vi "3_AC_Akım.vi"(10 "Ölçüm Süresi [sn]":i32=60, 11 "Remote IP Address":string="10.1.21.134") -> (0 "error out":errorcluster, 2 "AC AKIM Tüm Fazlar":sgl[][](array[numeric]) format="%.6f")   [LabVIEW 2014]
panel:
  in  "AC Akım FD2 Ic Register":u16=677
  in  "AC Akım FD2 Ib Register":u16=675
  in  "AC Akım FD2 Ia Register":u16=673
  out "AC Akım FD2 Ia":sgl[](array[numeric]) format="%_6f"
  out "AC Akım FD2 Ib":sgl[](array[numeric]) format="%_6f"
  out "AC Akım FD2 Ic":sgl[](array[numeric]) format="%_6f"
  out "AC Akım FD1 Ic":sgl[](array[numeric]) format="%_6f"
  out "AC Akım FD1 Ib":sgl[](array[numeric]) format="%_6f"
  out "AC Akım FD1 Ia":sgl[](array[numeric]) format="%_6f"
  in  "AC Akım FD1 Ic Register":u16=13
  in  "AC Akım FD1 Ib Register":u16=11
  out "Numeric":i32
  in  "AC Akım FD1 Ia Register":u16=9
  out "time stamp":timestamp=timestamp(1426515300 s since 1904-01-01) format="%<%H:%M:%S>T"
  in  "Remote Port":u16=1502
  in  "Stop":bool
  # "MB Ethernet Example Master.vi\n\nInstructions\n1. Run MB Ethernet Example Slave.vi\n2. Run this VI.\n3. Modify the discrete inputs or input registers on the slave -> they're updated on the master.\n4. Modify the coils and registers on the master -> they're updated on the slave."
  # "TCP Parameters"
  # "Slave Read-only Registers"
  # "FD1 Ia"
  # "FD1 Ib"
  # "FD1 Ic"
  # "FD2 Ia"
  # "FD2 Ib"
  # "FD2 Ic"
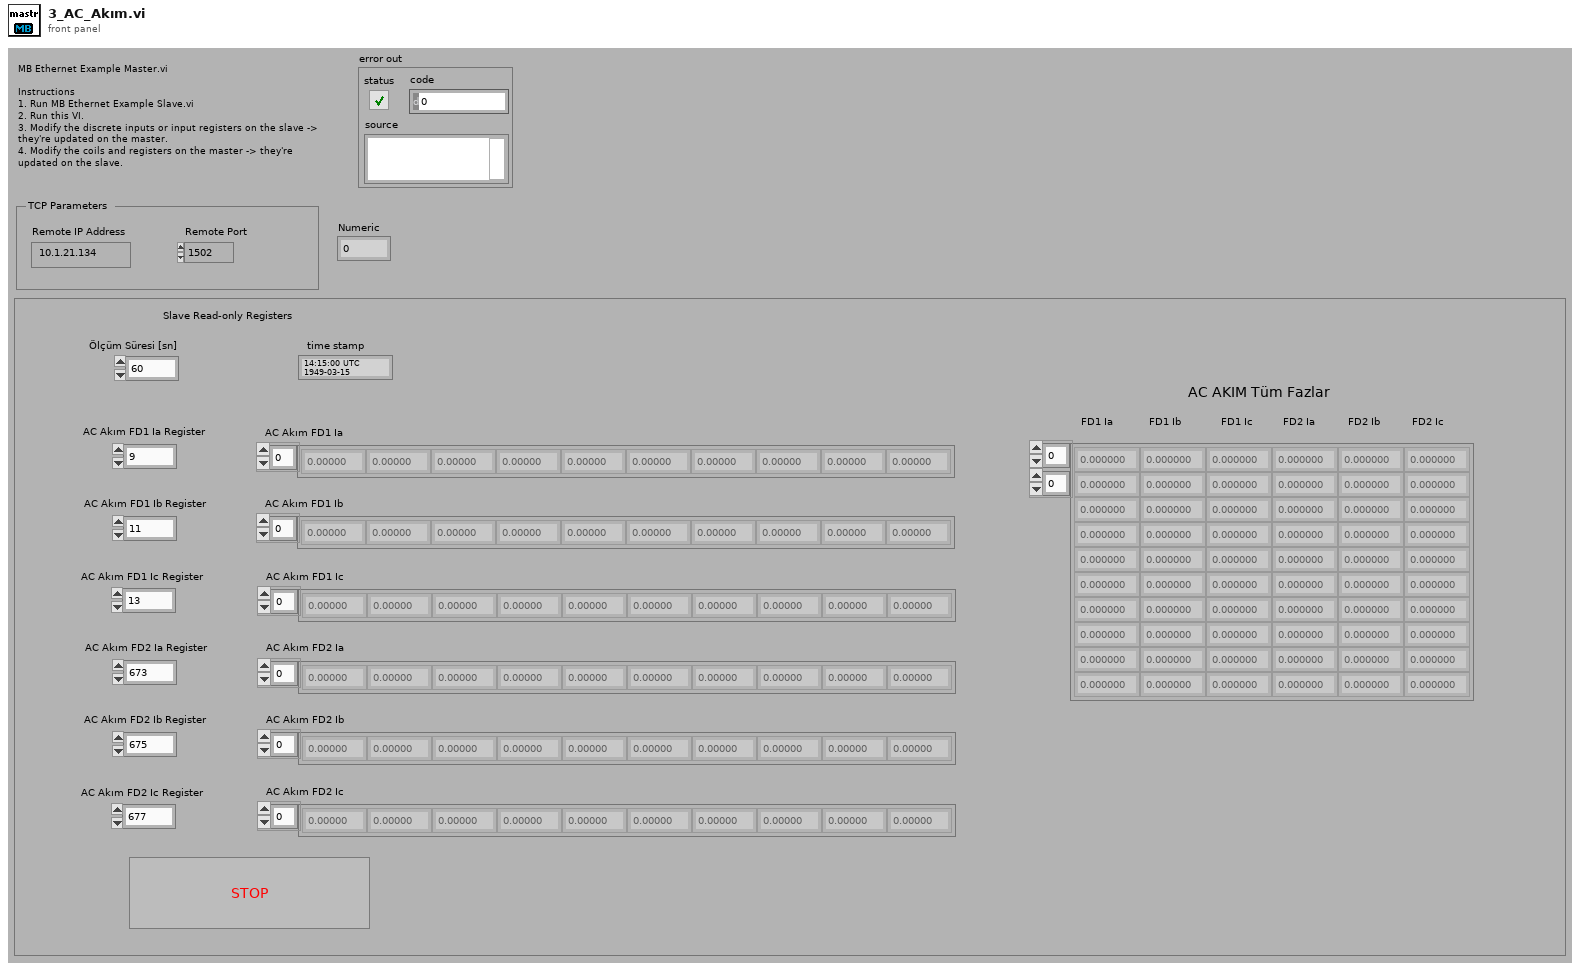
[diagram p1: front panel]
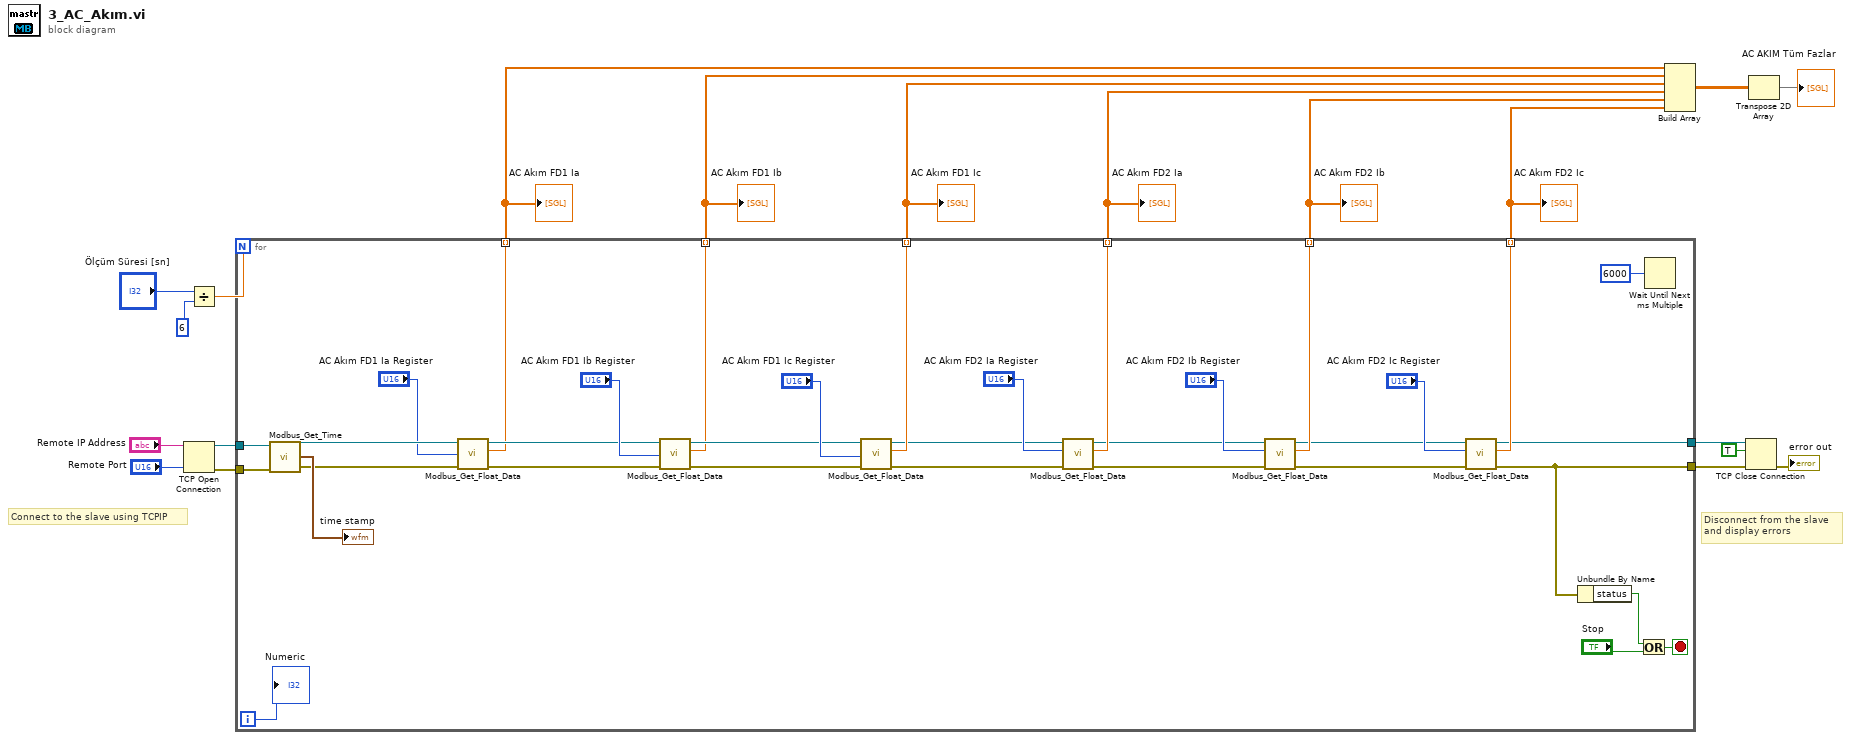
[diagram p0: block diagram]
diagram:
  # "Disconnect from the slave\nand display errors"
  # "Connect to the slave using TCPIP"
  n1 = TCP Open Connection(address="Remote IP Address", remote port or service name="Remote Port") -> (connection ID=w17:refnum<k5>, error out=w16:errorcluster)  [unwired: 1 in, 2 out]
  n2 = Divide(x="Ölçüm Süresi [sn]", y=6) -> (x/y=w12:dbl)
  n3 = for {
    N: w12 -> [_]
    tunnel: [w26] -> w15
    tunnel: w17 -> [w51]
    tunnel: w16 -> [w50]
    tunnel: [w22] -> w9
    tunnel: [w30] -> w8 mode=indexing
    tunnel: [w21] -> w7 mode=indexing
    tunnel: [w37] -> w6 mode=indexing
    tunnel: [w31] -> w5 mode=indexing
    tunnel: [w33] -> w4 mode=indexing
    tunnel: [w32] -> w3 mode=indexing
    i -> [w45]
    stop <- w20 stop-if-true
    n4 = call "Modbus_Get_Time.vi"("error in (no error)"=w50, "TCP Network Connection in"=w51) -> ("error out"=w46:errorcluster, "Time Stamp"=→"time stamp":timestamp, "TCP Network Connection out"=w48:refnum<k5>)  [unwired: 6 in, 1 out]
    n5 = call "Modbus_Get_Float_Data.vi"("error in (no error)"=w46, "Starting Address (2 Bytes)"="AC Akım FD1 Ia Register", "TCP Network Connection in"=w48) -> ("error out"=w42:errorcluster, "Numeric"=w30:sgl, "TCP Network Connection out"=w41:refnum<k5>)  [unwired: 5 in, 1 out]
    n6 = call "Modbus_Get_Float_Data.vi"("error in (no error)"=w42, "Starting Address (2 Bytes)"="AC Akım FD1 Ib Register", "TCP Network Connection in"=w41) -> ("error out"=w39:errorcluster, "Numeric"=w21:sgl, "TCP Network Connection out"=w38:refnum<k5>)  [unwired: 5 in, 1 out]
    n7 = call "Modbus_Get_Float_Data.vi"("error in (no error)"=w39, "Starting Address (2 Bytes)"="AC Akım FD1 Ic Register", "TCP Network Connection in"=w38) -> ("error out"=w29:errorcluster, "Numeric"=w37:sgl, "TCP Network Connection out"=w25:refnum<k5>)  [unwired: 5 in, 1 out]
    n8 = call "Modbus_Get_Float_Data.vi"("error in (no error)"=w29, "Starting Address (2 Bytes)"="AC Akım FD2 Ia Register", "TCP Network Connection in"=w25) -> ("error out"=w28:errorcluster, "Numeric"=w31:sgl, "TCP Network Connection out"=w24:refnum<k5>)  [unwired: 5 in, 1 out]
    n9 = call "Modbus_Get_Float_Data.vi"("error in (no error)"=w28, "Starting Address (2 Bytes)"="AC Akım FD2 Ib Register", "TCP Network Connection in"=w24) -> ("error out"=w27:errorcluster, "Numeric"=w33:sgl, "TCP Network Connection out"=w23:refnum<k5>)  [unwired: 5 in, 1 out]
    n10 = call "Modbus_Get_Float_Data.vi"("error in (no error)"=w27, "Starting Address (2 Bytes)"="AC Akım FD2 Ic Register", "TCP Network Connection in"=w23) -> ("error out"=w26:errorcluster, "Numeric"=w32:sgl, "TCP Network Connection out"=w22:refnum<k5>)  [unwired: 5 in, 1 out]
    n11 = Unbundle By Name(w26) -> ("status"=w52:bool)
    n12 = Or(x=w52, y="Stop") -> (x .or. y?=w20:bool)
    n13 = Wait Until Next ms Multiple(millisecond multiple=u32 6000) -> ()  [unwired: 1 out]
    "Numeric" <- w45
  }
  "AC Akım FD1 Ia" <- w8
  "AC Akım FD1 Ib" <- w7
  "AC Akım FD1 Ic" <- w6
  "AC Akım FD2 Ia" <- w5
  "AC Akım FD2 Ib" <- w4
  "AC Akım FD2 Ic" <- w3
  n14 = Build Array "Build Array"(w8, w7, w6, w5, w4, w3) -> (w2:sgl[][])
  n15 = TCP Close Connection(connection ID=w9, abort (F)=TRUE, error in (no error)=w15) -> (error out=→"error out":errorcluster)  [unwired: 1 out]
  n16 = Transpose 2D Array(2D array=w2) -> (transposed array=→"AC AKIM Tüm Fazlar":sgl[][])
